vi "Agilent U2000 Series Configure Gamma Table.vi"() -> ()   [LabVIEW 2018]
doc: "This example shows how to configure frequency and magnitude phase pairs for gamma table, and enable it.\n\nNote:\nThis VI is applicable for U2040 X-Series only."
uses:
  Agilent U2000 Series.lvlib
panel:
  in  "Enable Gamma Correction (T: Enable)":bool=TRUE
  in  "Magnitude Phase Pairs":dbl[](array[numeric])
  in  "Frequency Table Data":i32[](array[numeric])
  in  "Gamma Table Name (\"DEFAULT\")":string="DEFAULT"
  out "Measurement":dbl
  in  "VISA resource name":refnum<visa-resource-name>
  # "(c) 2011-2015 National Instruments.  ALL RIGHTS RESERVED."
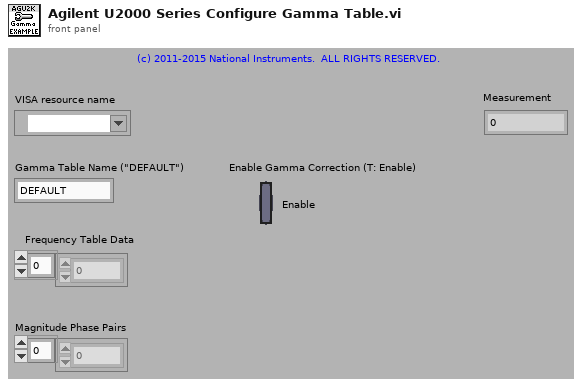
[diagram p1: front panel]
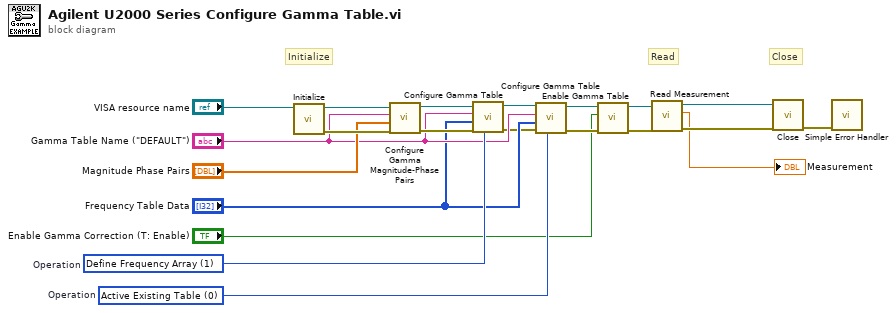
[diagram p0: block diagram]
diagram:
  w11 = 0 items=["Active Existing Table"=0, "Define Frequency Array"=1, "Rename Existing Table"=3, "Clear Existing Table"=4]  # Operation
  w15 = 1 items=["Active Existing Table"=0, "Define Frequency Array"=1, "Rename Existing Table"=3, "Clear Existing Table"=4]  # Operation
  # "Close"
  # "Read"
  # "Initialize"
  n1 = call "Initialize.vi"("VISA resource name"="VISA resource name") -> ("error out"=w19:errorcluster, "VISA resource name out"=w20:refnum<visa-resource-name>)  [unwired: 7 in, 2 out]
  n2 = call "Configure Gamma Magnitude-Phase Pairs.vi"("error in (no error)"=w19, "Magnitude Phase Pairs"="Magnitude Phase Pairs", "Gamma Table Name (\"DEFAULT\")"="Gamma Table Name (\"DEFAULT\")", "VISA resource name"=w20) -> ("error out"=w16:errorcluster, "VISA resource name out"=w17:refnum<visa-resource-name>)  [unwired: 6 in]
  n3 = call "Configure Gamma Table.vi"("Operation (0: Active Existing Table)"=w15, "error in (no error)"=w16, "Table Data"="Frequency Table Data", "Gamma Table Name (\"DEFAULT\")"="Gamma Table Name (\"DEFAULT\")", "VISA resource name"=w17) -> ("error out"=w6:errorcluster, "VISA resource name out"=w14:refnum<visa-resource-name>)  [unwired: 5 in]
  n4 = call "Configure Gamma Table.vi"("Operation (0: Active Existing Table)"=w11, "error in (no error)"=w6, "Table Data"="Frequency Table Data", "Gamma Table Name (\"DEFAULT\")"="Gamma Table Name (\"DEFAULT\")", "VISA resource name"=w14) -> ("error out"=w7:errorcluster, "VISA resource name out"=w8:refnum<visa-resource-name>)  [unwired: 5 in]
  n5 = call "Enable Gamma Table.vi"("error in (no error)"=w7, "Enable Gamma Correction (T: Enable)"="Enable Gamma Correction (T: Enable)", "VISA resource name"=w8) -> ("error out"=w10:errorcluster, "VISA resource name out"=w9:refnum<visa-resource-name>)  [unwired: 7 in]
  n6 = call "Read Measurement.vi"("error in (no error)"=w10, "VISA resource name"=w9) -> ("error out"=w3:errorcluster, "Measurement"=→"Measurement":dbl, "VISA resource name out"=w4:refnum<visa-resource-name>)  [unwired: 1 in, 6 out]
  n7 = call "Close.vi"("error in (no error)"=w3, "VISA resource name"=w4) -> ("error out"=w2:errorcluster)  [unwired: 9 out]
  n8 = call <vilib>:"Simple Error Handler.vi"("error in (no error)"=w2) -> ()  [unwired: 1 in, 8 out]
